vi "Compute ScanLimits.vi"(8 "error in (no error)":errorcluster, 9 "Samples Per Inch":i32, 10 "Inspect Start Axial Position":dbl, 11 "Inspect Axial Length":dbl) -> (0 "error out":errorcluster, 1 "PosToStartScan(Cnts)":i32, 2 "ScanLength(Cnts)":i32, 3 "PosToEndScan(Cnts)":i32, 5 "Max Samples":i32)   [LabVIEW 2015, in "Tool Module.lvlib"]
doc: "<b>Note:</b> This VI was modified by the <b>Validate DQMH Module</b> tool to turn off automatic error handling."
uses:
  Tool Module.lvlib
  Tool Config/Tool Cfg.lvlib
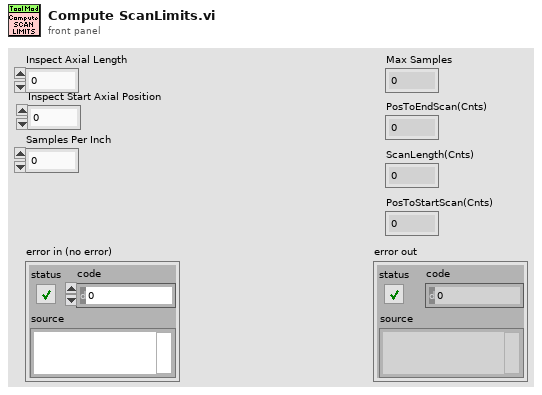
[diagram p1: front panel]
types:
  T1 = typedef "Tool Module.lvlib/Get-Set Inspection Limits (Reply Payload)--cluster.ctl" = cluster{"Inspection Limits":T2, "Get-Set Inspection Limits_error":errorcluster}
  T2 = typedef "Tool Module.lvlib/_Inspection Limits cluster--typedef.ctl" = cluster{"MaxSamples":i32, "PosToStartScan":i32, "PosToEndScan":i32, "ScanLength":i32}
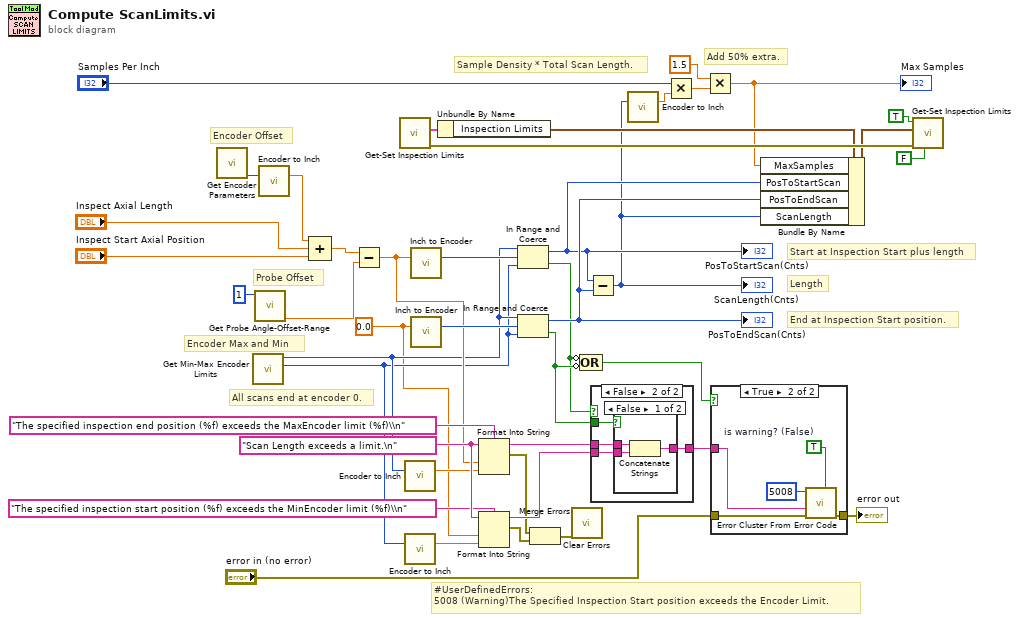
[diagram p0: block diagram]
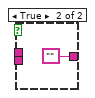
[diagram p3: hidden frame]
diagram:
  w4 = 0.0 ("input 1")
  w26 = "Scan Length exceeds a limit.\n" ("error message (\"\")")
  # "All scans end at encoder 0."
  # "Sample Density * Total Scan Length."
  # "Add 50% extra."
  # "Encoder Max and Min"
  # "Probe Offset"
  # "Encoder Offset"
  # "#UserDefinedErrors:\n5008 (Warning)The Specified Inspection Start position exceeds the Encoder Limit."
  # "End at Inspection Start position."
  # "Length"
  # "Start at Inspection Start plus length"
  n1 = call "Get Encoder Parameters.vi"() -> ("Encoder Offset"=w16:i32)  [unwired: 9 in, 2 out]
  n2 = call "Get Min-Max Encoder Limits.vi"() -> ("MinEncoder"=w14:i32, "MaxEncoder"=w15:i32)  [unwired: 8 in, 2 out]
  n3 = call "Get Probe Angle-Offset-Range.vi"("Probe Select"=1) -> ("Probe Offset"=w12:sgl)  [unwired: 7 in, 3 out]
  n4 = call "Encoder to Inch.vi"("Encoder in"=w16) -> ("Encoder out(in)"=w18:dbl)  [unwired: 14 in]
  n5 = Compound Arithmetic op=ADD(w18, "Inspect Axial Length", "Inspect Start Axial Position") -> (w40:dbl)
  n6 = Subtract(x=w40, y=w12) -> (x-y=w17:dbl)
  n7 = call "Get-Set Inspection Limits.vi"() -> ("error out"=w41:errorcluster, "Reply Payload"=w1:T1)  [unwired: 9 in, 1 out]
  n8 = call "Encoder to Inch.vi"("Encoder in"=w15) -> ("Encoder out(in)"=w22:dbl)  [unwired: 14 in]
  n9 = call "Encoder to Inch.vi"("Encoder in"=w14) -> ("Encoder out(in)"=w21:dbl)  [unwired: 14 in]
  n10 = call "Inch to Encoder.vi"("Inches in"=w17) -> ("Encoder out"=w43:i32)  [unwired: 14 in]
  n11 = call "Inch to Encoder.vi"("Inches in"=w4) -> ("Encoder out"=w42:i32)  [unwired: 14 in]
  n12 = Unbundle By Name(w1) -> ("Inspection Limits"=w20:T2)
  n13 = Format Into String(format string="The specified inspection end position (%f) exceeds the MaxEncoder limit (%f)\\n" ("error message (\"\")"), initial string=w26, w17, w22) -> (resulting string=w31:string, error out=w28:errorcluster)  [unwired: 1 in]
  n14 = Format Into String(format string="The specified inspection start position (%f) exceeds the MinEncoder limit (%f)\\n" ("error message (\"\")"), initial string=w26, w4, w21) -> (resulting string=w32:string, error out=w29:errorcluster)  [unwired: 1 in]
  n15 = In Range and Coerce(upper limit=w15, x=w43, lower limit=w14) -> (coerced(x)=w38:i32, In Range?=w33:bool)
  "PosToStartScan(Cnts)" <- w38
  n16 = In Range and Coerce(upper limit=w15, x=w42, lower limit=w14) -> (coerced(x)=w39:i32, In Range?=w34:bool)
  "PosToEndScan(Cnts)" <- w39
  n17 = Merge Errors(w28, w29) -> (w30:errorcluster)
  n18 = call <vilib>:"Clear Errors.vi"("error in (no error)"=w30) -> ()  [unwired: 5 in, 2 out]
  n19 = Compound Arithmetic op=OR(invert w33, invert w34) -> (w23:bool)
  n20 = Subtract(x=w38, y=w39) -> (x-y=w10:i32)
  "ScanLength(Cnts)" <- w10
  n21 = case shown="False" w33 {
    tunnel: w31 -> [w47 w53]
    tunnel: w32 -> [w46 w52]
    tunnel: w34 -> [w45 w51]
    tunnel: [w44 w50] -> w35
    frame True {
      n22 = case shown="False" w45 {
        tunnel: w47 -> [_ _]
        tunnel: w46 -> [w48 _]
        tunnel: [w48 ""] -> w44
        frame False {
        }
        frame True {
        }
      }
    }
    frame False {
      n23 = case shown="False" w51 {
        tunnel: w53 -> [w54 w57]
        tunnel: w52 -> [w55 _]
        tunnel: [w56 w57] -> w50
        frame False {
          n24 = Concatenate Strings(w54, w55) -> (w56:string)
        }
        frame True {
        }
      }
    }
  }
  n25 = call "Encoder to Inch.vi"("Encoder in"=w10) -> ("Encoder out(in)"=w9:dbl)  [unwired: 14 in]
  n26 = Multiply(x="Samples Per Inch", y=w9) -> (x*y=w8:dbl)
  n27 = Multiply(x=1.5, y=w8) -> (x*y=w7:dbl)
  "Max Samples" <- w7
  n28 = case shown="True" w23 {
    tunnel: "error in (no error)" -> [w58 w63]
    tunnel: [w58 w62] -> w36
    tunnel: w35 -> [_ w59]
    frame False {
    }
    frame True {
      w61 = TRUE  # is warning? (False)
      n29 = call <vilib>:"Error Cluster From Error Code.vi"("is warning? (False)"=w61, "error in (no error)"=w63, "error message (\"\")"=w59, "error code (0)"=5008) -> ("error out"=w62:errorcluster)  [unwired: 5 in]
    }
  }
  "error out" <- w36
  n30 = Bundle By Name(cluster=w20, "MaxSamples"=w7, "PosToStartScan"=w38, "PosToEndScan"=w39, "ScanLength"=w10) -> (w19:T2)
  n31 = call "Get-Set Inspection Limits.vi"("wait for reply (T)"=FALSE, "error in (no error)"=w41, "Inspection Limits"=w19, "Set"=TRUE) -> ()  [unwired: 5 in, 3 out]
